vi "Verify Telemetry Session is Idle.vi"(0 "error in":errorcluster, 1 "poll delay (500 ms)":dbl[unit]=0.5, 2 "max attempts (10)":i32=10, 3 "VISA resource":refnum<visa-resource-name>="COM13") -> (7 "error out":errorcluster, 9 "idle":bool)   [LabVIEW 2010]
doc: "This function polls the Telemetry base station multiple times, until the base station status is idle or a time-out."
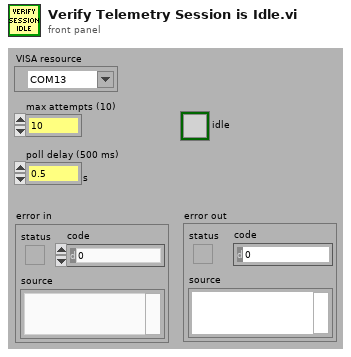
[diagram p1: front panel]
types:
  T1 = cluster{"ERROR_OCCURRED":bool, "LINK_STAT_CHANGED":bool, "LINK_QUAL_CHANGED":bool, "400MHZ_TX_ACTIVE":bool, "400MHZ_RX_ACTIVE":bool, "245GHZ_TX_ACTIVE":bool, "DATA_STAT_CHANGED":bool, "SLEEPING":bool, "IDLE":bool, "SEARCHING_FOR_IMPLANT":bool, "STARTING_SESSION":bool, "LISTENING_FOR_EMERG":bool, "IN_SESSION":bool}
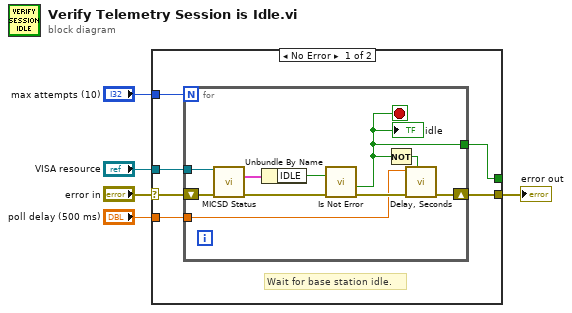
[diagram p0: block diagram]
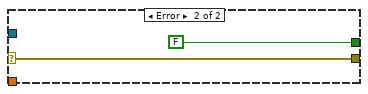
[diagram p2: hidden frame]
diagram:
  n1 = case shown="No Error" "error in" {
    selector: "error in" -> [w8 w23]
    tunnel: "VISA resource" -> [w11 _]
    tunnel: "max attempts (10)" -> [w10 _]
    tunnel: "poll delay (500 ms)" -> [w9 _]
    tunnel: [w7 w23] -> w1
    tunnel: [w6 FALSE ("ready")] -> _
    frame No Error {
      # "Wait for base station idle."
      n2 = for {
        N: w10 -> [_]
        tunnel: w11 -> [w20]
        tunnel: [w14] -> w6
        tunnel: w9 -> [w13]
        shift-right: [w16] -> w7
        shift-left: w8 -> [w12]
        stop <- w14 stop-if-true
        n3 = call "MICSD Status.vi"("VISA Resource Name"=w20, "error in (no error)"=w12) -> ("Status Flags"=w21:T1, "error out"=w19:errorcluster)  [unwired: 7 in, 5 out]
        n4 = Unbundle By Name(w21) -> ("IDLE"=w17:bool)
        n5 = call "Is Not Error.vi"("enable (T)"=w17, "error in"=w19) -> ("error out"=w18:errorcluster, "ready"=w14:bool)  [unwired: 4 in, 1 out]
        "idle" <- w14
        n6 = Not(x=w14) -> (.not. x?=w15:bool)
        n7 = call "Delay, Seconds.vi"("enable (T)"=w15, "error in"=w18, "delay"=w13) -> ("error out"=w16:errorcluster)  [unwired: 4 in, 1 out]
      }
    }
    frame Error {
    }
  }
  "error out" <- w1
